vi "Create RS-xxx.vi"(8 "error in (no error)":errorcluster, 9 "PCL Decimation":u16, 10 "Protocol Properties":T3, 11 "Target in":refnum<k24>) -> (0 "error out":errorcluster, 1 "Message Channels refnums":T2 {"Enable Periodic" format="%.0x"; "Error Code" format="%.0x"; "Message Status" format="%.0x"; "Timestamp" format="%.0x"; "Trigger" format="%.0x"}, 2 "Instrument Addon Custom Device refnum":T1=18446744073709551615 format="%.0x", 3 "Target out":refnum<k24>)   [LabVIEW 2019, in "Scripting API.lvlib"]
uses:
  Scripting API.lvlib
  NationalInstruments.VeriStand.SystemDefinitionAPI
  <vilib>/NI VeriStand/Custom Device API/Custom Device Item Ref.ctl
  <vilib>/NI VeriStand/Custom Device API/Custom Device API.lvlib
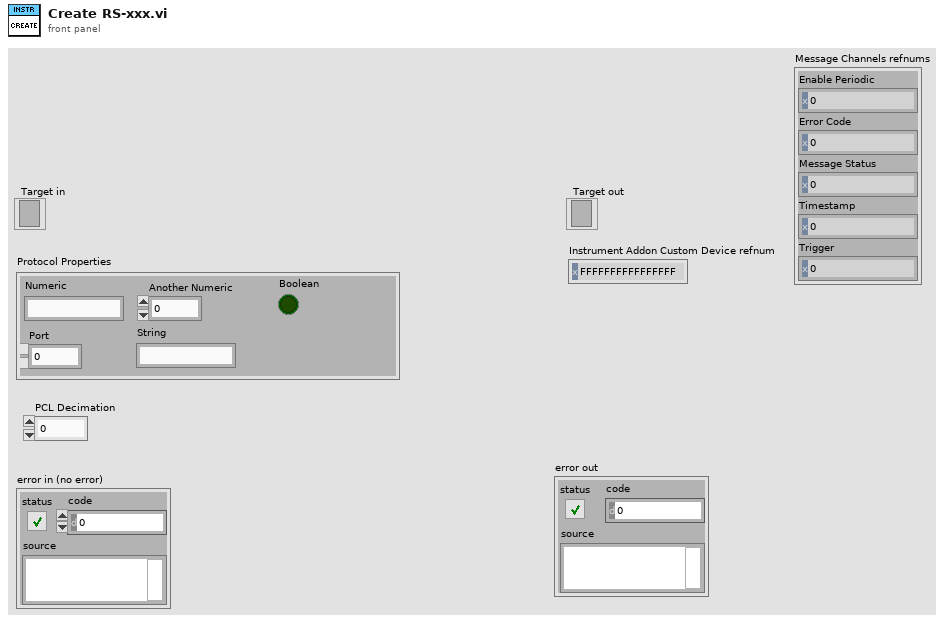
[diagram p1: front panel]
types:
  T1 = typedef "Custom Device API.lvlib/Custom Device Item Ref.ctl" = u64
  T2 = cluster{"Enable Periodic":T1, "Error Code":T1, "Message Status":T1, "Timestamp":T1, "Trigger":T1}
  T3 = cluster{"Numeric":string, "Port":dbl, "Another Numeric":dbl, "Boolean":bool, "String":string}
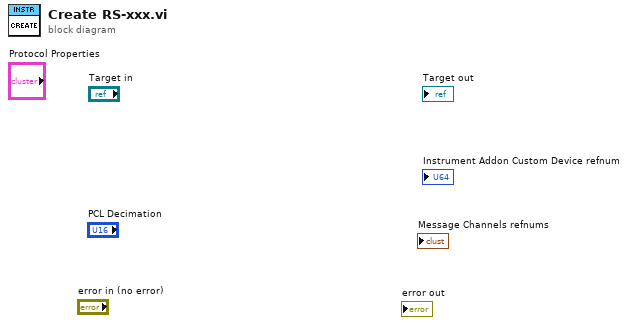
[diagram p0: block diagram]
diagram:
